vi "food.vi"() -> ()   [LabVIEW 2016]
panel:
  in  "PIZZA":string="PIZZA"
  out "AMOUNT":dbl
  out "ORDER STATUS":string
  in  "?":string="FOODIES STALL"
  out "BILL":dbl
  out "output cluster":T1 caption="ORDER LIST"
  in  "CFF":string="COFFEE"
  in  "SW":string="SANWICH "
  in  "BR":string="BRIYANI"
  in  "BL":string="B.L CHICKEN"
  in  "CK":string="COKE"
  in  "CL":string="CHICKEN LEGS"
  in  "CW":string="CHICKEN WINGS"
  in  "FF":string="FRENCH FRIES"
  in  "BURGER":string="BURGER"
  in  "ITEM":bool caption="ITEM1"
  in  "QUANTITY":dbl=1.0 min=1.0 max=10.0 step=1.0
  out "PRICE":dbl=100.0
  in  "ITEM 2":bool caption="ITEM1"
  in  "QUANTITY 2":dbl=1.0 min=1.0 max=10.0 step=1.0
  out "PRICE 2":dbl=200.0
  in  "ITEM 3":bool caption="ITEM1"
  in  "QUANTITY 3":dbl=1.0 min=1.0 max=10.0 step=1.0
  out "PRICE 3":dbl=150.0
  in  "ITEM 4":bool caption="ITEM1"
  in  "QUANTITY4":dbl=1.0 min=1.0 max=10.0 step=1.0
  out "PRICE 4":dbl=250.0
  in  "ITEM 5":bool caption="ITEM1"
  in  "QUANTITY 5":dbl=1.0 min=1.0 max=10.0 step=1.0
  out "PRICE 5":dbl=225.0
  out "Discount":string
  in  "OK Button":bool
  in  "ITEM 6":bool caption="ITEM1"
  in  "QUANTITY 6":dbl=1.0 min=1.0 max=10.0 step=1.0
  in  "ITEM 7":bool caption="ITEM1"
  in  "QUANTITY 7":dbl=1.0 min=1.0 max=10.0 step=1.0
  in  "ITEM 8":bool caption="ITEM1"
  in  "QUANTITY 8":dbl=1.0 min=1.0 max=10.0 step=1.0
  in  "ITEM 9":bool caption="ITEM1"
  in  "QUANTITY 9":dbl=1.0 min=1.0 max=10.0 step=1.0
  in  "ITEM 10":bool caption="ITEM1"
  in  "QUANTITY 10":dbl=1.0 min=1.0 max=10.0 step=1.0
  out "PRICE 10":dbl=25.0
  out "PRICE 7":dbl=350.0
  out "PRICE 6":dbl=50.0
  out "PRICE 8":dbl=380.0
  out "PRICE 9":dbl=180.0
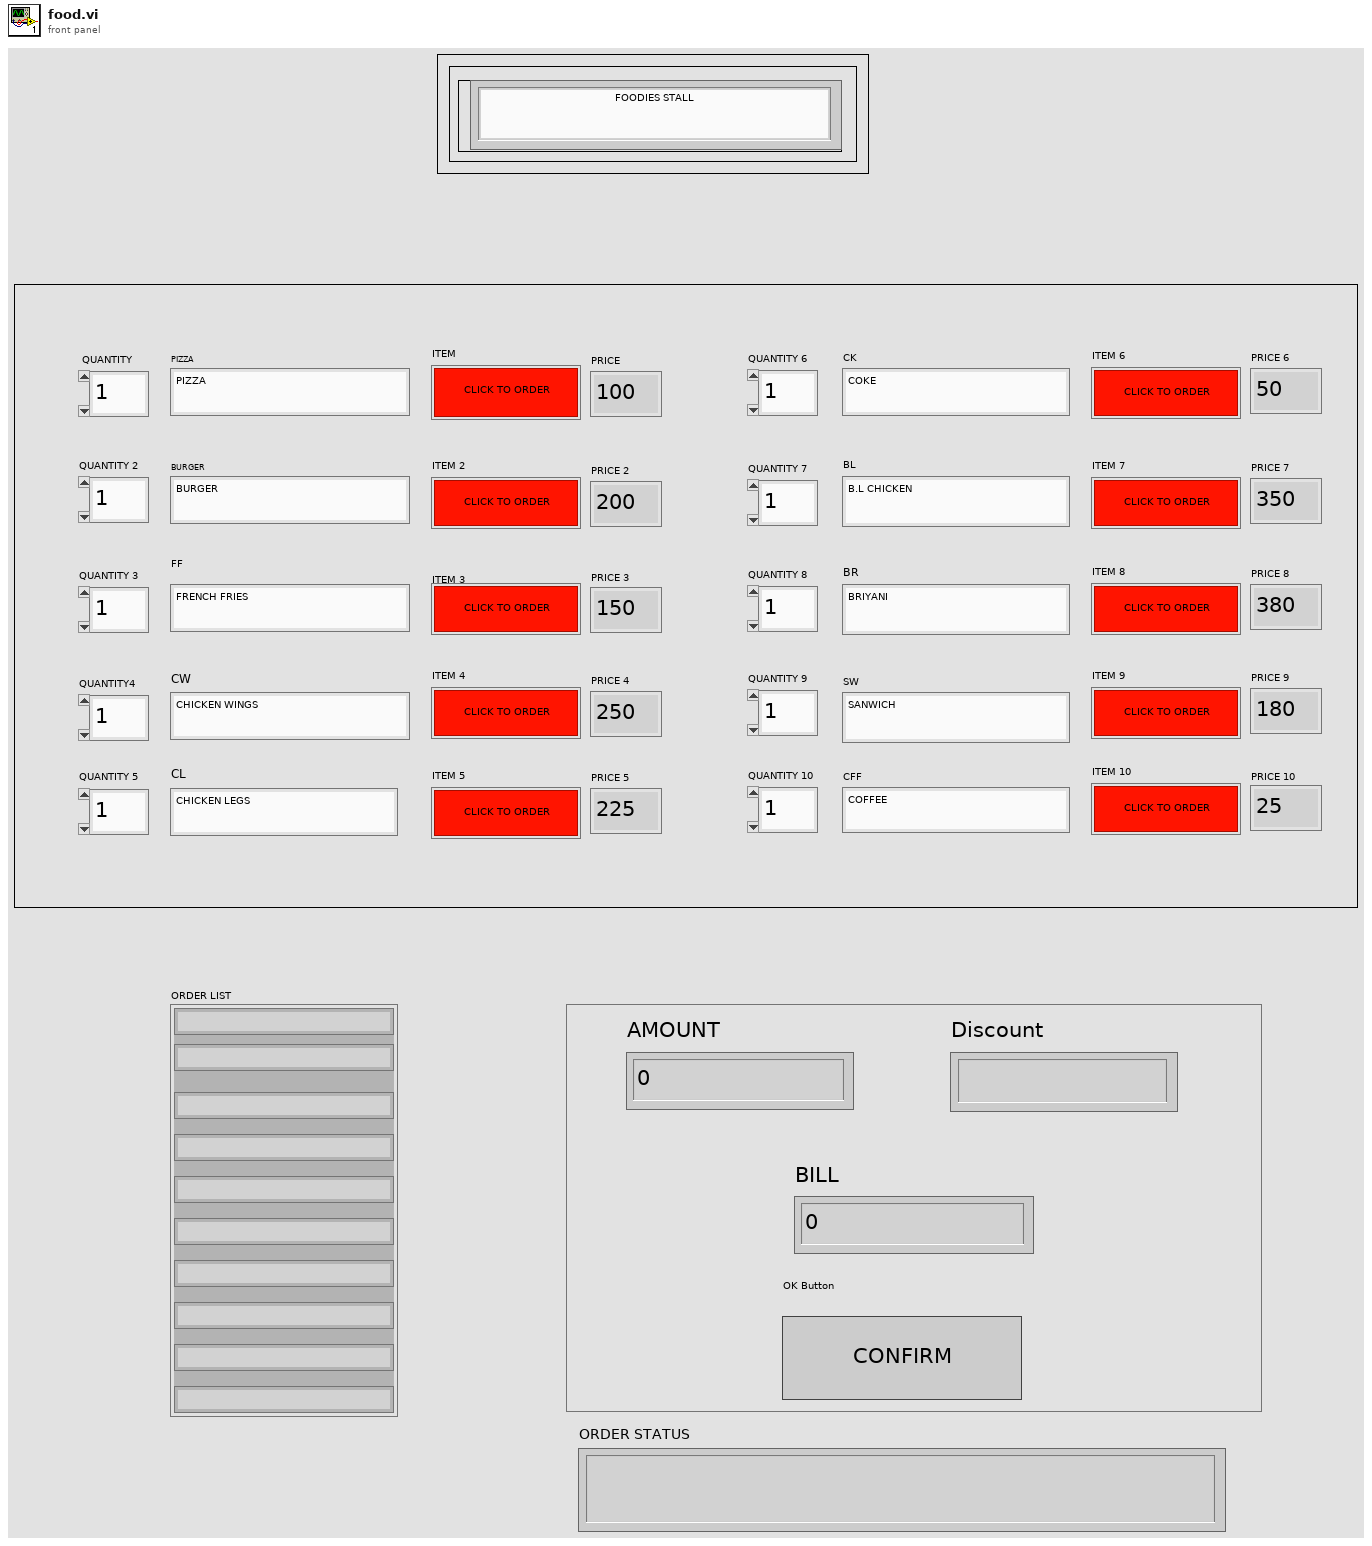
[diagram p1: front panel]
types:
  T1 = cluster{string, string, string, string, string, string, string, string, string, string}
  T2 = cluster{"sanwich":string, "boneless":string, "legs":string, "wings":string, "puffs":string, "briyani":string, "coke":string, "pizza":string, "burger":string, "french fries":string}
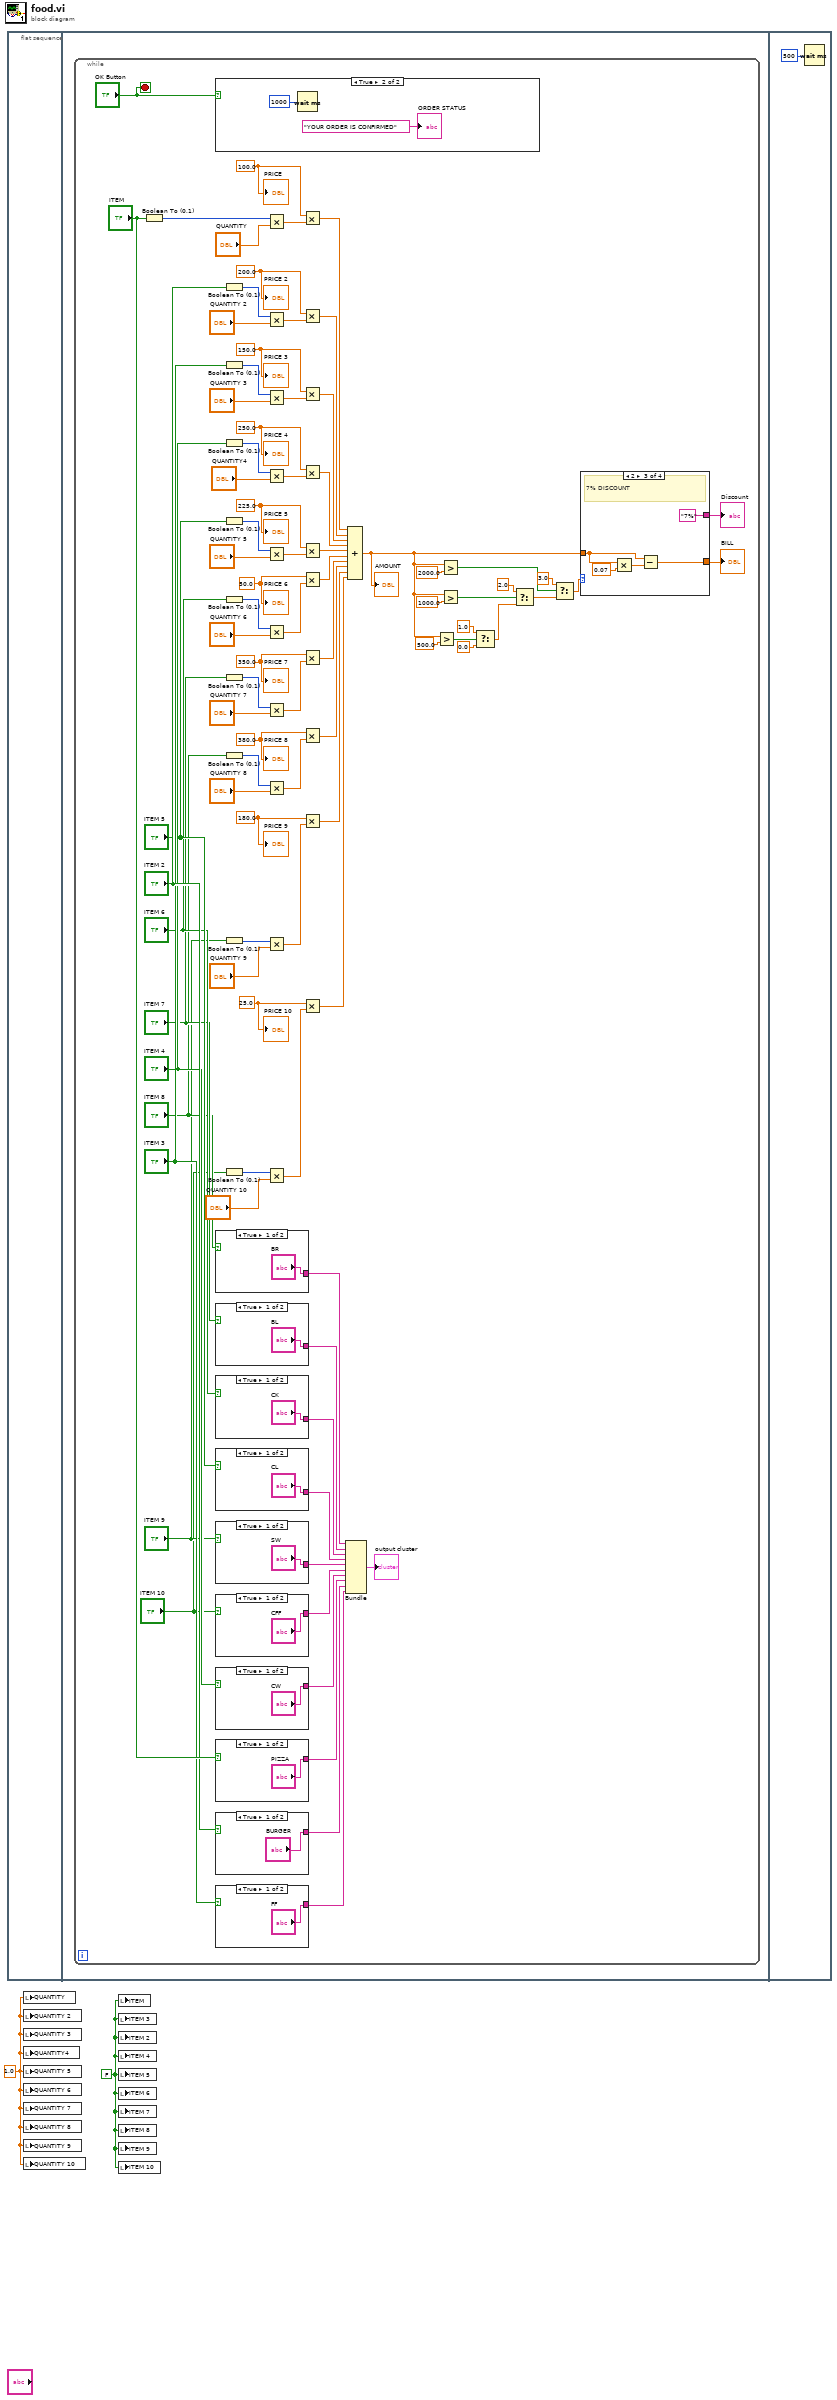
[diagram p0: block diagram]
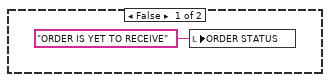
[diagram p2: hidden frame]
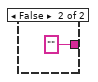
[diagram p3: hidden frame]
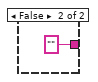
[diagram p4: hidden frame]
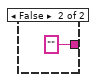
[diagram p5: hidden frame]
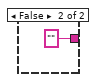
[diagram p6: hidden frame]
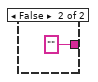
[diagram p7: hidden frame]
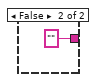
[diagram p8: hidden frame]
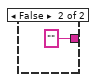
[diagram p9: hidden frame]
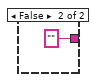
[diagram p10: hidden frame]
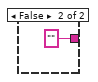
[diagram p11: hidden frame]
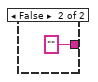
[diagram p12: hidden frame]
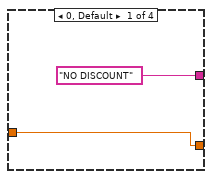
[diagram p13: hidden frame]
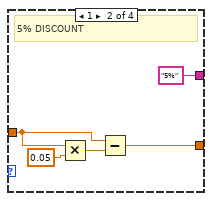
[diagram p14: hidden frame]
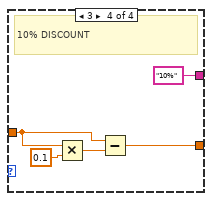
[diagram p15: hidden frame]
diagram:
  w1 = 1.0 ("QUANTITY4")
  w2 = FALSE ("ITEM 5")
  n1 = flat-sequence {
    frame #0 {
    }
    frame #1 {
      n2 = while {
        stop <- "OK Button" stop-if-true
        w27 = 25.0 ("PRICE")
        w29 = 180.0 ("PRICE")
        w31 = 380.0 ("PRICE")
        w33 = 350.0 ("PRICE")
        w34 = 50.0 ("PRICE")
        w72 = 225.0 ("PRICE")
        w76 = 250.0 ("PRICE")
        w80 = 150.0 ("PRICE")
        w84 = 200.0 ("PRICE")
        w88 = 100.0 ("PRICE")
        n3 = Boolean To (0,1)(Boolean="ITEM") -> (0, 1=w90:i16)
        n4 = case shown="True" "OK Button" {
          frame False {
            n5 = local write "ORDER STATUS"("ORDER IS YET TO RECEIVE" ("ORDER STATUS")) -> ()
          }
          frame True {
            n6 = Wait (ms)(milliseconds to wait=u32 1000) -> ()  [unwired: 1 out]
            "ORDER STATUS" <- "YOUR ORDER IS CONFIRMED"
          }
        }
        n7 = case shown="True" "ITEM 8" {
          tunnel: ["BR" "" ("sanwich")] -> w16
          frame True {
          }
          frame False {
          }
        }
        n8 = case shown="True" "ITEM 7" {
          tunnel: ["BL" "" ("boneless")] -> w17
          frame True {
          }
          frame False {
          }
        }
        n9 = case shown="True" "ITEM 6" {
          tunnel: ["CK" "" ("legs")] -> w18
          frame True {
          }
          frame False {
          }
        }
        n10 = case shown="True" "ITEM 5" {
          tunnel: ["CL" "" ("wings")] -> w19
          frame True {
          }
          frame False {
          }
        }
        n11 = case shown="True" "ITEM 9" {
          tunnel: ["SW" "" ("puffs")] -> w20
          frame True {
          }
          frame False {
          }
        }
        n12 = case shown="True" "ITEM 10" {
          tunnel: ["CFF" "" ("briyani")] -> w21
          frame True {
          }
          frame False {
          }
        }
        n13 = case shown="True" "ITEM 4" {
          tunnel: ["CW" "" ("coke")] -> w22
          frame True {
          }
          frame False {
          }
        }
        n14 = case shown="True" "ITEM" {
          tunnel: ["PIZZA" "" ("pizza")] -> w25
          frame True {
          }
          frame False {
          }
        }
        n15 = case shown="True" "ITEM 2" {
          tunnel: ["BURGER" "" ("burger")] -> w24
          frame True {
          }
          frame False {
          }
        }
        n16 = case shown="True" "ITEM 3" {
          tunnel: ["FF" "" ("french fries")] -> w23
          frame True {
          }
          frame False {
          }
        }
        n17 = Boolean To (0,1)(Boolean="ITEM 2") -> (0, 1=w86:i16)
        n18 = Boolean To (0,1)(Boolean="ITEM 3") -> (0, 1=w82:i16)
        n19 = Boolean To (0,1)(Boolean="ITEM 4") -> (0, 1=w78:i16)
        n20 = Boolean To (0,1)(Boolean="ITEM 5") -> (0, 1=w74:i16)
        n21 = Boolean To (0,1)(Boolean="ITEM 6") -> (0, 1=w50:i16)
        n22 = Boolean To (0,1)(Boolean="ITEM 7") -> (0, 1=w47:i16)
        n23 = Boolean To (0,1)(Boolean="ITEM 8") -> (0, 1=w45:i16)
        n24 = Boolean To (0,1)(Boolean="ITEM 9") -> (0, 1=w43:i16)
        n25 = Boolean To (0,1)(Boolean="ITEM 10") -> (0, 1=w41:i16)
        n26 = Multiply(x=w90, y="QUANTITY") -> (x*y=w87:dbl)
        n27 = Multiply(x=w86, y="QUANTITY 2") -> (x*y=w83:dbl)
        n28 = Multiply(x=w82, y="QUANTITY 3") -> (x*y=w79:dbl)
        n29 = Multiply(x=w78, y="QUANTITY4") -> (x*y=w75:dbl)
        n30 = Multiply(x=w74, y="QUANTITY 5") -> (x*y=w71:dbl)
        n31 = Multiply(x=w50, y="QUANTITY 6") -> (x*y=w49:dbl)
        n32 = Multiply(x=w47, y="QUANTITY 7") -> (x*y=w46:dbl)
        n33 = Multiply(x=w45, y="QUANTITY 8") -> (x*y=w44:dbl)
        n34 = Multiply(x=w43, y="QUANTITY 9") -> (x*y=w42:dbl)
        n35 = Multiply(x=w41, y="QUANTITY 10") -> (x*y=w40:dbl)
        n36 = Multiply(x=w88, y=w87) -> (x*y=w70:dbl)
        n37 = Multiply(x=w84, y=w83) -> (x*y=w69:dbl)
        n38 = Multiply(x=w80, y=w79) -> (x*y=w68:dbl)
        n39 = Multiply(x=w76, y=w75) -> (x*y=w67:dbl)
        n40 = Multiply(x=w72, y=w71) -> (x*y=w66:dbl)
        n41 = Multiply(x=w34, y=w49) -> (x*y=w48:dbl)
        n42 = Multiply(x=w33, y=w46) -> (x*y=w39:dbl)
        n43 = Multiply(x=w31, y=w44) -> (x*y=w38:dbl)
        n44 = Multiply(x=w29, y=w42) -> (x*y=w37:dbl)
        n45 = Multiply(x=w27, y=w40) -> (x*y=w36:dbl)
        n46 = Bundle("sanwich"=w16, "boneless"=w17, "legs"=w18, "wings"=w19, "puffs"=w20, "briyani"=w21, "coke"=w22, "pizza"=w25, "burger"=w24, "french fries"=w23) -> (→"output cluster":T2)  [unwired: 1 in]
        n47 = Compound Arithmetic op=ADD(w70, w69, w68, w67, w66, w48, w39, w38, w37, w36) -> (w53:dbl)
        "AMOUNT" <- w53
        n48 = Greater?(x=w53, y=500.0) -> (0:w62:bool)
        n49 = Greater?(x=w53, y=2000.0) -> (0:w60:bool)
        n50 = Greater?(x=w53, y=1000.0) -> (0:w61:bool)
        n51 = Select(t=1.0, s=w62, f=0.0) -> (s? t:f=w55:dbl)
        n52 = Select(t=2.0, s=w61, f=w55) -> (s? t:f=w54:dbl)
        n53 = Select(t=3.0, s=w60, f=w54) -> (s? t:f=w51:dbl)
        n54 = case shown="2" w51 {
          tunnel: [w115 w117 w122 w128] -> w5
          tunnel: w53 -> [w115 w118 w123 w127]
          tunnel: ["NO DISCOUNT" ("Discount") "5%" ("Discount") "7%" ("Discount") "10%" ("Discount")] -> w52
          frame 0, Default {
          }
          frame 1 {
            # "5% DISCOUNT"
            n55 = Multiply(x=w118, y=0.05) -> (x*y=w119:dbl)
            n56 = Subtract(x=w118, y=w119) -> (x-y=w117:dbl)
          }
          frame 2 {
            # "7% DISCOUNT"
            n57 = Multiply(x=w123, y=0.07) -> (x*y=w125:dbl)
            n58 = Subtract(x=w123, y=w125) -> (x-y=w122:dbl)
          }
          frame 3 {
            # "10% DISCOUNT"
            n59 = Multiply(x=w127, y=0.1) -> (x*y=w130:dbl)
            n60 = Subtract(x=w127, y=w130) -> (x-y=w128:dbl)
          }
        }
        "Discount" <- w52
        "BILL" <- w5
        "PRICE" <- w88
        "PRICE 2" <- w84
        "PRICE 3" <- w80
        "PRICE 4" <- w76
        "PRICE 5" <- w72
        "PRICE 10" <- w27
        "PRICE 7" <- w33
        "PRICE 6" <- w34
        "PRICE 8" <- w31
        "PRICE 9" <- w29
      }
    }
    frame #2 {
      n61 = Wait (ms)(milliseconds to wait=u32 500) -> ()  [unwired: 1 out]
    }
  }
  n62 = local write "QUANTITY"(w1) -> ()
  n63 = local write "QUANTITY 2"(w1) -> ()
  n64 = local write "QUANTITY 3"(w1) -> ()
  n65 = local write "QUANTITY4"(w1) -> ()
  n66 = local write "QUANTITY 5"(w1) -> ()
  n67 = local write "QUANTITY 6"(w1) -> ()
  n68 = local write "QUANTITY 7"(w1) -> ()
  n69 = local write "QUANTITY 8"(w1) -> ()
  n70 = local write "QUANTITY 9"(w1) -> ()
  n71 = local write "QUANTITY 10"(w1) -> ()
  n72 = local write "ITEM"(w2) -> ()
  n73 = local write "ITEM 3"(w2) -> ()
  n74 = local write "ITEM 2"(w2) -> ()
  n75 = local write "ITEM 4"(w2) -> ()
  n76 = local write "ITEM 5"(w2) -> ()
  n77 = local write "ITEM 6"(w2) -> ()
  n78 = local write "ITEM 7"(w2) -> ()
  n79 = local write "ITEM 8"(w2) -> ()
  n80 = local write "ITEM 9"(w2) -> ()
  n81 = local write "ITEM 10"(w2) -> ()
